vi "GenRandom.vi"(7 "MaxColor":u32(colorbox), 11 "NumLeds":i32) -> (3 "Array":u32[](array[numeric]))   [LabVIEW 2025, in "ArduinoSerialBling.lvlib"]
uses:
  ArduinoSerialBling.lvlib
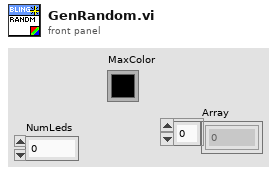
[diagram p1: front panel]
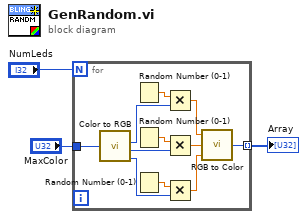
[diagram p0: block diagram]
diagram:
  n1 = for {
    N: "NumLeds" -> [_]
    tunnel: [w8] -> w3 mode=indexing
    tunnel: "MaxColor" -> [w4]
    n2 = call <vilib>:"Color to RGB.vi"("Color"=w4) -> ("R"=w7:u8, "G"=w6:u8, "B"=w5:u8)  [unwired: 1 out]
    n3 = Random Number (0-1)() -> (number: 0 to 1=w14:dbl)
    n4 = Random Number (0-1)() -> (number: 0 to 1=w11:dbl)
    n5 = Random Number (0-1)() -> (number: 0 to 1=w10:dbl)
    n6 = Multiply(x=w14, y=w7) -> (x*y=w13:dbl)
    n7 = Multiply(x=w11, y=w6) -> (x*y=w12:dbl)
    n8 = Multiply(x=w10, y=w5) -> (x*y=w9:dbl)
    n9 = call <vilib>:"RGB to Color.vi"("B"=w9, "G"=w12, "R"=w13) -> ("Color"=w8:u32)
  }
  "Array" <- w3
